vi "PWM POC.vi"() -> ()   [LabVIEW 2014]
uses:
  Public/Utilities/Open Local.vi
  Public/Peripherals/PWM/PWM Set Duty Cycle N Chans.vi
  LMH-LINX.lvlib
panel:
  in  "Stop Button":bool
  in  "PWM Channels":u8[](array[numeric])=[13, 19, 60, 62]
  in  "Duty Cycles":dbl[](array[numeric])=[0.25, 0.5, 0.75, 1.0]
  out "Error Out":errorcluster
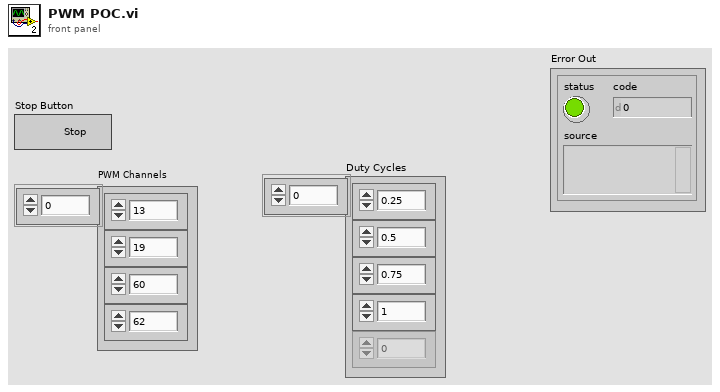
[diagram p1: front panel]
types:
  T1 = typedef "LMH-LINX.lvlib/LINX Ref.ctl" = cluster{"IO":T2, "Interface":T3, "LINX Device Config":T4}
  T2 = typedef "LMH-LINX.lvlib/Platform.ctl" = enum16{"Remote", "Local"}
  T3 = typedef "LMH-LINX.lvlib/Interface.ctl" = enum16{"Serial", "TCP"}
  T4 = typedef "LMH-LINX.lvlib/Device.lvlib/LINX Device Config.ctl" = cluster{"Interface":T3, "COM Port":refnum<visa-resource-name>, "TCP Configuration":T5, "Device Family":u8, "Device ID":u8, "Device Name":string, "TCP Ref":refnum<k5>, "Channels":T6}
  T5 = typedef "LMH-LINX.lvlib/Device.lvlib/TCP Config.ctl" = cluster{"IP Address":string, "Port":u16}
  T6 = typedef "LMH-LINX.lvlib/Channels.ctl" = cluster{"DI":u8[], "DO":u8[], "AI":u8[], "AO":u8[], "PWM":u8[], "QE":u8[], "UART":u8[], "I2C 2":u8[], "SPI":u8[], "CAN":u8[], "Servo":u8[], "AI Ref (V)":dbl, "AI Resolution (Bits)":u8, "AO Ref (V)":dbl, "AO Resolution (Bits)":u8}
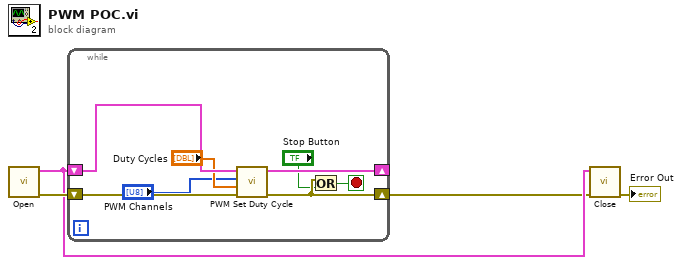
[diagram p0: block diagram]
diagram:
  n1 = call-poly "Open.vi"() -> ("Error Out"=w4:errorcluster, "LINX Resource"=w2:T1)  [unwired: 9 in, 1 out]
  n2 = while {
    shift-right: [w11] -> _
    shift-left: w2 -> [w12]
    shift-right: [w8] -> w1
    shift-left: w4 -> [w10]
    stop <- w9 stop-if-true
    n3 = call-poly "PWM Set Duty Cycle.vi"("Error In"=w10, "Duty Cycles"="Duty Cycles", "PWM Channels"="PWM Channels", "LINX Resource"=w12) -> ("Error Out"=w8:errorcluster, "LINX Resource"=w11:T1)  [unwired: 6 in]
    n4 = Or(x=w8, y="Stop Button") -> (x .or. y?=w9:bool)
  }
  n5 = call "Close.vi"("Error In"=w1, "LINX Resource"=w2) -> ("Error Out"=→"Error Out":errorcluster)  [unwired: 9 in]
